vi "IRISS V2 XYZ Ref Follow.vi"(5 "Left or Right Arm":i32(ring)=1 items=["Left Arm", "Right Arm"], 6 "error in":errorcluster, 7 "Accurus Ctrl Cluster":T2={"Stop Vacuum"=TRUE, "Vacuum Force"=0, "Max Limit [mmHg]"=600.0, "Slide in"=0, "Irrigation?"=TRUE} {"Slide in" scale=0.0..78.0; "Vacuum Force" min=0 max=78}, 8 "XYZ Cmd Posit":dbl[](array[numeric]), 9 "FPGA VI Reference In":refnum<k20>) -> (0 "error out":errorcluster, 1 "Accurus Output Cluster":T1, 2 "XYZ Out Posit":dbl[](array[numeric]), 3 "FPGA VI Reference Out":refnum<k20>)   [LabVIEW 2016]
uses:
  EyeRobotDLL.dll
  <vilib>/rvi/interface/nirviReadWriteControl/nirviReadWriteControl.xnode
  FPGA Bitfiles/PhantomControlPI_FPGATarget_QuadCtr2_E2412E44.lvbitx
  IRISS_FPGA_IO.vi
  NiFpgaLv.dll
  <vilib>/Utility/error.llb/Error Cluster From Error Code.vi
  <vilib>/rvi/errors/niLvFpgaAdjustHostInterfaceError.vi
panel:
  out "grasp":dbl
  # "button 1"
  # "button 2"
  # "button 3"
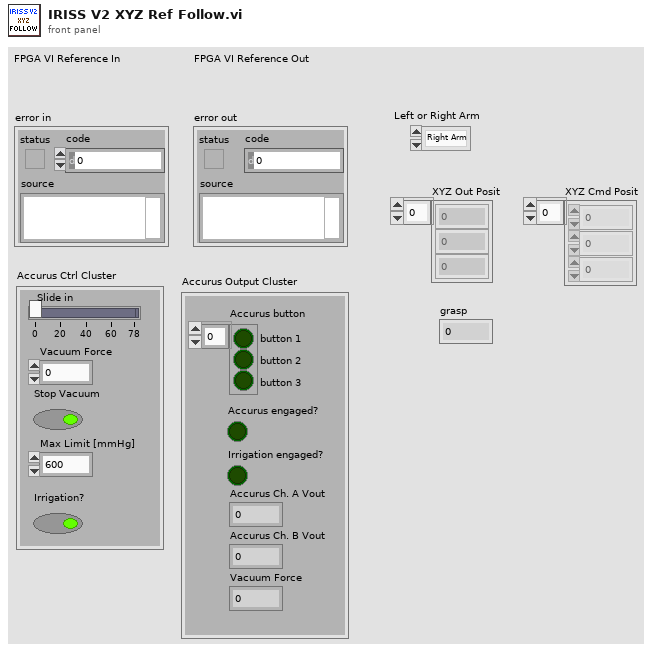
[diagram p1: front panel]
types:
  T1 = cluster{"Accurus button":bool[], "Accurus engaged?":bool, "Vacuum Force":i32, "Accurus Ch. A Vout":dbl, "Accurus Ch. B Vout":dbl, "Irrigation engaged?":bool}
  T2 = cluster{"Stop Vacuum":bool, "Vacuum Force":i8, "Max Limit [mmHg]":dbl, "Slide in":i8, "Irrigation?":bool}
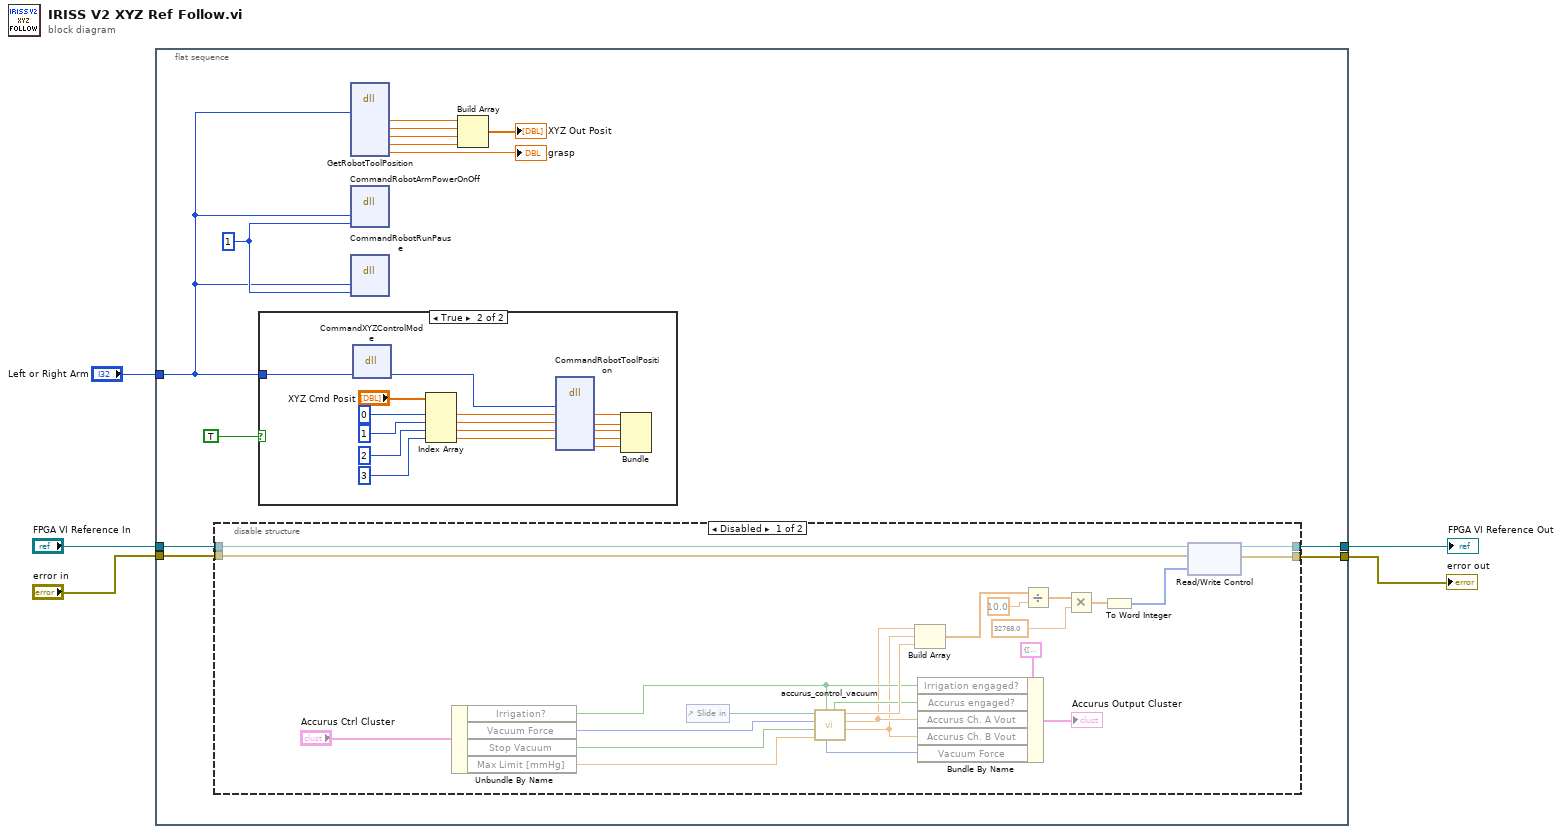
[diagram p0: block diagram]
diagram:
  n1 = flat-sequence {
    tunnel: "Left or Right Arm" -> [w6]
    tunnel: "FPGA VI Reference In" -> [w10]
    tunnel: "error in" -> [w9]
    tunnel: [w8] -> w3
    tunnel: [w7] -> w2
    frame #0 {
      w17 = 1 ("OnOff")
      n2 = disable-structure shown="Disabled" {
        disable-tunnel: w10 -> [w22 _]
        disable-tunnel: w9 -> [w21 _]
        disable-tunnel: [w20 _] -> w8
        disable-tunnel: [w19 _] -> w7
        frame Disabled {
          n3 = Unbundle By Name("Accurus Ctrl Cluster") -> ("Irrigation?"=w34:bool, "Vacuum Force"=w39:i8, "Stop Vacuum"=w38:bool, "Max Limit [mmHg]"=w37:dbl)
          n4 = control-ref of="Slide in"() -> (w36:refnum<vi>)
          n5 = call "accurus_control_vacuum.vi"("Irrigate?"=w34, "Max Limit [mmHg]"=w37, "stop"=w38, "vacuum force"=w39, "Slide in"=w36) -> ("f"=w31:dbl, "f 2"=w32:dbl, "f 3"=w41:dbl, "Boolean 2"=w33:bool, "Vacuum Force\n[mmHg]"=w30:i32)  [unwired: 1 in, 1 out]
          n6 = Build Array(w32, w31, w41) -> (w24:dbl[])
          n7 = Bundle By Name(cluster=T1 {"Accurus button"=[FALSE, FALSE, FALSE], "Accurus engaged?"=FALSE, "Vacuum Force"=0, "Accurus Ch. A Vout"=0.0, "Accurus Ch. B Vout"=0.0, "Irrigation engaged?"=FALSE} ("Accurus Output Cluster"), "Irrigation engaged?"=w34, "Accurus engaged?"=w33, "Accurus Ch. A Vout"=w32, "Accurus Ch. B Vout"=w31, "Vacuum Force"=w30) -> (→"Accurus Output Cluster":T1)
          n8 = Divide(x=w24, y=10.0) -> (x/y=w26:dbl[])
          n9 = Multiply(x=w26, y=32768.0) -> (x*y=w28:dbl[])
          n10 = To Word Integer(number=w28) -> (16bit integer=w23:i16[])
          n11 = xnode "Read/Write Control"("FPGA VI Reference In"=w22, "error in"=w21, "AO"=w23) -> ("FPGA VI Reference Out"=w20:refnum<k20>, "error out"=w19:errorcluster)
        }
        frame Enabled {
        }
      }
      n12 = case shown="True" TRUE {
        tunnel: w6 -> [_ w57]
        frame False {
        }
        frame True {
          n13 = dll-call lib="D:/IRISSoft LV2016 beta/Host Demo/Functions/EyeRobotDLL.dll" fn="CommandXYZControlMode"("id"=w57) -> ("id"=w51:i32)  [unwired: 4 in, 2 out]
          n14 = Index Array(array="XYZ Cmd Posit", index #1=0 ("index"), index #2=1 ("index"), index #3=2 ("index"), index #4=3 ("index")) -> (element #1=w47:dbl, element #2=w46:dbl, element #3=w44:dbl, element #4=w43:dbl)
          n15 = dll-call lib="D:/IRISSoft LV2016 beta/Host Demo/Functions/EyeRobotDLL.dll" fn="CommandRobotToolPosition"("id"=w51, "x"=w47, "y"=w46, "z"=w44, "roll"=w43) -> ("x"=w56:dbl, "y"=w55:dbl, "z"=w54:dbl, "roll"=w53:dbl, "grasp"=w52:dbl)  [unwired: 6 in, 2 out]
          n16 = Bundle("x"=w56, "y"=w55, "z"=w54, "roll"=w53, "grasp"=w52) -> ()  [unwired: 1 in, 1 out]
        }
      }
      n17 = dll-call lib="D:/IRISSoft LV2016 beta/Host Demo/Functions/EyeRobotDLL.dll" fn="GetRobotToolPosition"("id"=w6) -> ("x"=w16:dbl, "y"=w14:dbl, "z"=w15:dbl, "roll"=w13:dbl, "grasp"=→"grasp":dbl)  [unwired: 10 in, 2 out]
      n18 = dll-call lib="D:/IRISSoft LV2016 beta/Host Demo/Functions/EyeRobotDLL.dll" fn="CommandRobotArmPowerOnOff"("id"=w6, "OnOff"=w17) -> ()  [unwired: 6 in, 2 out]
      n19 = dll-call lib="D:/IRISSoft LV2016 beta/Host Demo/Functions/EyeRobotDLL.dll" fn="CommandRobotRunPause"("id"=w6, "RunPause"=w17) -> ()  [unwired: 6 in, 2 out]
      n20 = Build Array(w16, w14, w15, w13) -> (→"XYZ Out Posit":dbl[])
    }
  }
  "error out" <- w2
  "FPGA VI Reference Out" <- w3
